vi "SystemTimeStamptoCVT.vi"(8 "error in (no error)":errorcluster, 11 "BaseDriver in":refnum<class "BaseDriver.lvclass">) -> (0 "error out":errorcluster, 3 "BaseDriver out":refnum<class "BaseDriver.lvclass">)   [LabVIEW 2020, in "BaseDriver.lvclass"]
doc: "This VI does 2 things - \n\n1. It updates a variable called system timestamp in the CVT\n2. If the scan is OFF and save is ON, the timestamp information is used to put into the filename.\n\nNOTE - If the custom timestamp is updated anywhere in the acquire case, that information is used for\nlabelling, if not then the systemtimestamp is used for labelling"
uses:
  BaseDriver.lvclass
  BaseDriver.lvclass/BaseDriver.ctl
  shared/CompressAndUpdate(Poly)/CompressAndUpdate(Numeric).vi
panel:
  out "SysTmestamp":dbl format="%.3f"
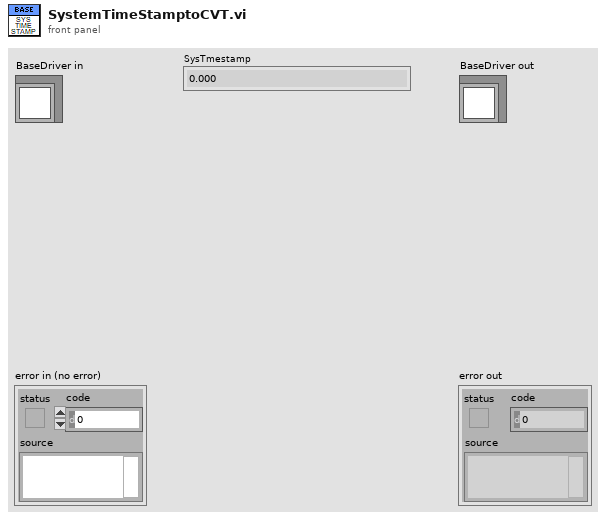
[diagram p1: front panel]
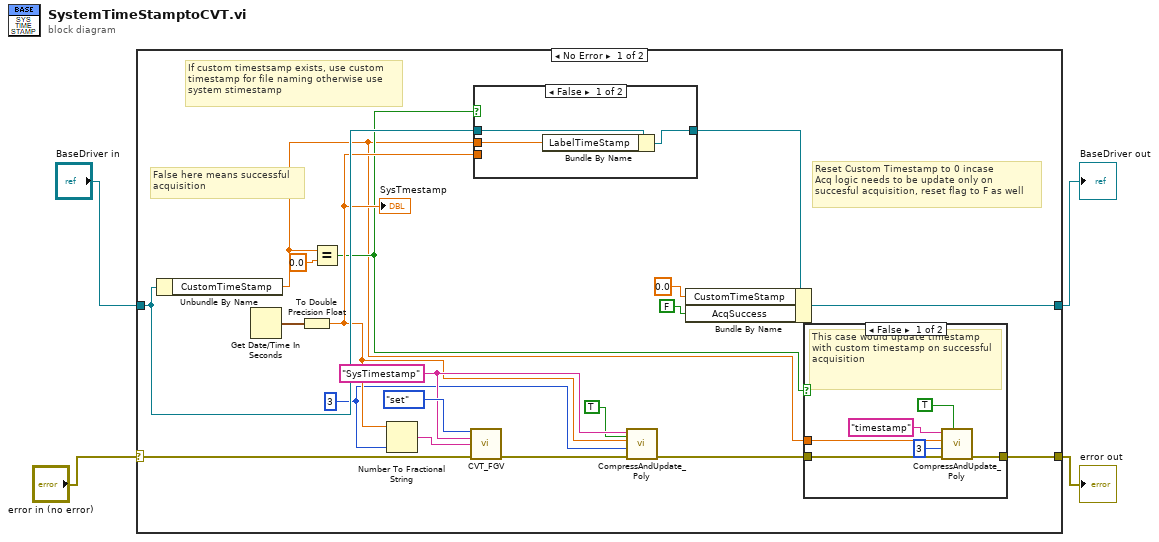
[diagram p0: block diagram]
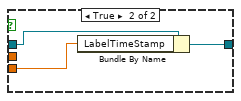
[diagram p3: hidden frame]
diagram:
  n1 = case shown="No Error" "error in (no error)" {
    selector: "error in (no error)" -> [w21 w38]
    tunnel: [w6 w38] -> w4
    tunnel: [w9 w37] -> w2
    tunnel: "BaseDriver in" -> [w18 w37]
    frame No Error {
      w13 = i16 3 ("precision (6)")
      w15 = "SysTimestamp" ("variable")
      # "False here means successful \nacquisition"
      # "Reset Custom Timestamp to 0 incase\nAcq logic needs to be update only on \nsuccesful acquisition, reset flag to F as well"
      # "If custom timestsamp exists, use custom\ntimestamp for file naming otherwise use\nsystem stimestamp"
      n2 = Unbundle By Name(w18) -> ("CustomTimeStamp"=w5:dbl)
      n3 = Get Date/Time In Seconds() -> (seconds since 1Jan1904=w23:timestamp)
      n4 = To Double Precision Float(number=w23) -> (double precision float=w14:dbl)
      "SysTmestamp" <- w14
      n5 = Equal?(x=w5, y=0.0) -> (x = y?=w11:bool)
      n6 = Number To Fractional String(number=w14, precision (6)=w13) -> (F-format string=w20:string)  [unwired: 2 in]
      n7 = call "CVT_FGV.vi"("command"=enum16{"set", "get", "reset", "get all"}."set", "variable"=w15, "value in"=w20, "error in"=w21) -> ("error out"=w16:errorcluster)  [unwired: 9 in, 2 out]
      n8 = case shown="False" w11 {
        tunnel: w18 -> [w32 w36]
        tunnel: w14 -> [_ w35]
        tunnel: [w33 w34] -> w10
        tunnel: w5 -> [w31 _]
        frame False {
          n9 = Bundle By Name(cluster=w32, "LabelTimeStamp"=w31) -> (w33:refnum<class "BaseDriver.lvclass">)
        }
        frame True {
          n10 = Bundle By Name(cluster=w36, "LabelTimeStamp"=w35) -> (w34:refnum<class "BaseDriver.lvclass">)
        }
      }
      n11 = call-poly "CompressAndUpdate_Poly.vi"("force CVT update (false)"=TRUE, "error in"=w16, "precision (6)"=w13, "Numeric"=w14, "command or variable name"=w15) -> ("error out"=w7:errorcluster)  [unwired: 6 in]
      n12 = Bundle By Name(cluster=w10, "CustomTimeStamp"=0.0 ("y"), "AcqSuccess"=FALSE) -> (w9:refnum<class "BaseDriver.lvclass">)
      n13 = case shown="False" w11 {
        tunnel: w7 -> [w28 w30]
        tunnel: [w27 w30] -> w6
        tunnel: w5 -> [w26 _]
        frame False {
          # "This case would update timestamp with custom timestamp on successful acquisition"
          n14 = call-poly "CompressAndUpdate_Poly.vi"("force CVT update (false)"=TRUE, "error in"=w28, "precision (6)"=i16 3, "Numeric"=w26, "command or variable name"="timestamp") -> ("error out"=w27:errorcluster)  [unwired: 6 in]
        }
        frame True {
        }
      }
    }
    frame Error {
    }
  }
  "error out" <- w4
  "BaseDriver out" <- w2
